vi "Edit VI Theme.vi"(10 "VI Refnum":refnum<vi>) -> ()   [LabVIEW 2021]
doc: "This VI will be the user interface function for the Quick Drop action or through the Tools Menu .\n\nIt will list: +\n- Theme File referenced by the VI (if saved as part of the User Tag data) +\n- Theme Mode referenced by the VI (if saved) +\n- Front Panel Color Rule +\n- All non-free-label Decorations and their color rules; organized by UID because that is the exposed property that is an identifier +\n- All controls on the front panel along with their Color Rules, Boolean Types (if applicable), and Tab Color (if applicable). This will be populated before showing its front panel and will give the user faster access to edit all controls on the front panel. +\n\n->Apply Deocration Rules to see the application of the change +\n->Apply Color Rules to see the application of changes to the controls on the FP +\n->Save VI in order to save all tag data (including theme file and mode reference) +\n\n<b>Code Developed By:</b> +\nDaniel Coons +\nTechnology Service Corporation +\nwww.tsc.com/atcs"
uses:
  Material Theme/Material Theme.lvclass
  _theme-editor/Theme Config/Theme Config.lvclass/Theme Config.ctl
  Material SubVIs/Material SubVIs.lvlib
  user32.dll
  _theme-editor/Theme Config/Theme Config.lvclass
  Quick Drop Plugins/TSC Control Theme Application.llb/control info--typedef.ctl
  Quick Drop Plugins/TSC Control Theme Application.llb/decorations info--typedef.ctl
panel:
  in  "decroation--apply":bool
  in  "decorations":T1[](array[typedef]) {"Decoration Level" items=["Undefined", "Default", "Surface", "Background", "Surface Dim", "Surface Variant", "Surface Bright", "Surface Container Lowest", "Surface Container Low", "Surface Container", "Surface Container High", "Surface Container Highest", "Inverse Surface"]}
  in  "Front Panel Rule":u16(ring) items=["Undefined", "Default", "Surface", "Background", "Surface Dim", "Surface Variant", "Surface Bright", "Surface Container Lowest", "Surface Container Low", "Surface Container", "Surface Container High", "Surface Container Highest", "Inverse Surface"]
  in  "Material Theme":refnum<class "Material Theme.lvclass">
  in  "Close":bool
  in  "save":bool
  in  "Theme Mode":u16(ring) items=["Light", "Light Medium Contrast", "Light High Contrast", "Dark", "Dark Medium Contrast", "Dark High Contrast"]
  in  "Path to theme file":path
  out "Name of VI":string
  in  "apply":bool
  out "header":bool
  in  "Controls":T2[](array[typedef]) {"tab level" items=["Undefined", "N/A", "Default", "Primary Container", "Secondary Container", "Tertiary Container", "Error Container", "Surface", "Background", "Surface Dim", "Surface Variant", "Surface Bright", "Surface Container Lowest", "Surface Container Low", "Surface Container", "Surface Container High", "Surface Container Highest", "Inverse Surface", "Inverse Primary"]; "Boolean Type" items=["Undefined", "N/A", "Outline", "No-Outline", "Tonal", "Filled", "Transparent", "FAB", "Elevated"]; "UI Theme Level" items=["Undefined", "N/A", "Primary", "Secondary", "Tertiary", "Error", "Primary Fixed", "Secondary Fixed", "Tertiary Fixed", "Label Only", "No Change"]}
  # "Decoration UID"
  # "Decoration Color Rule"
  # "Control Name"
  # "Data Type"
  # "Color Rule"
  # "Boolean Type"
  # "Tab Color"
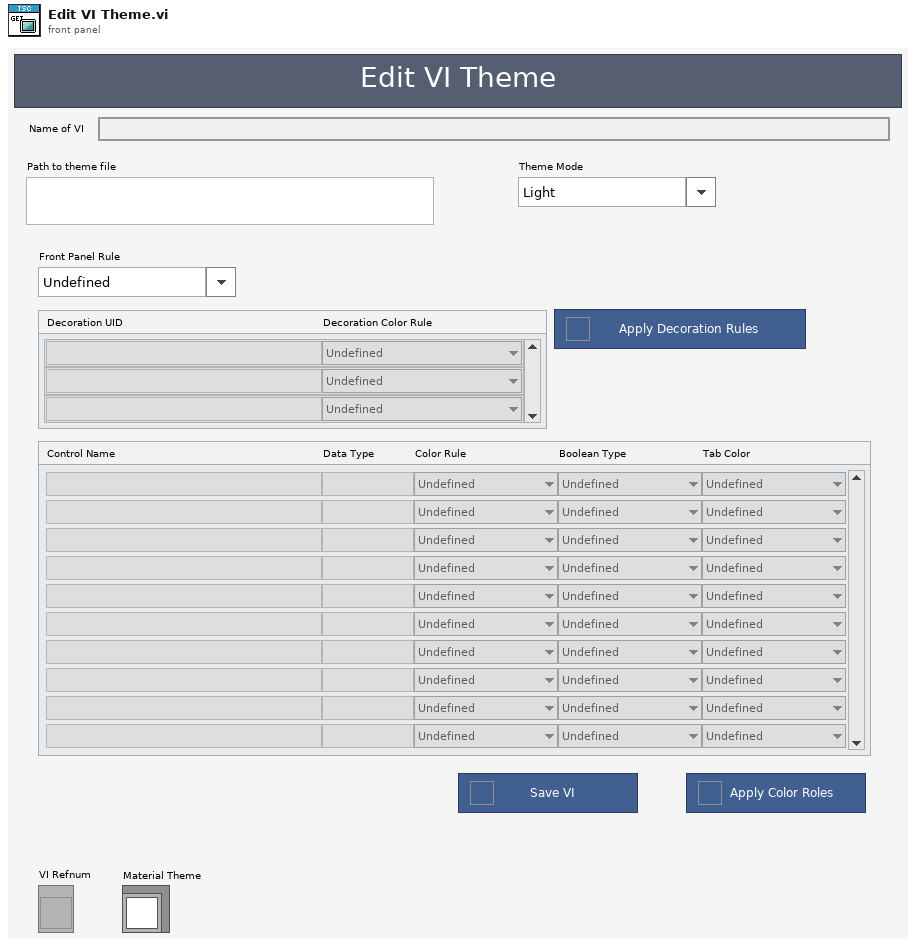
[diagram p1: front panel]
types:
  T1 = typedef "decorations info--typedef.ctl" = cluster{"label":string, "Decoration Level":u16}
  T2 = typedef "control info--typedef.ctl" = cluster{"label":string, "control type":string, "UI Theme Level":u16, "Boolean Type":u16, "tab level":u16}
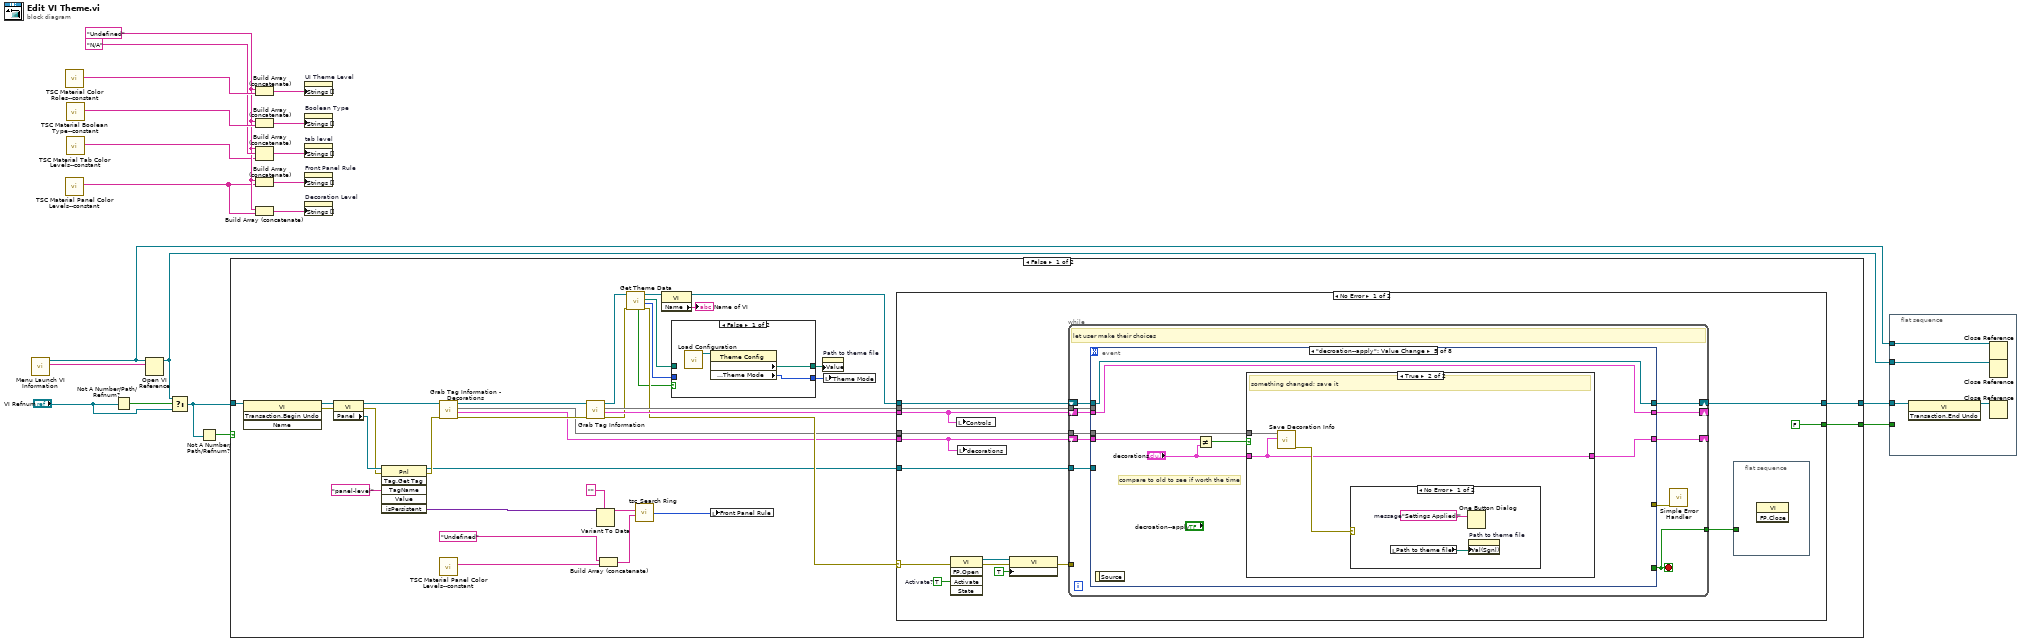
[diagram p0: block diagram]
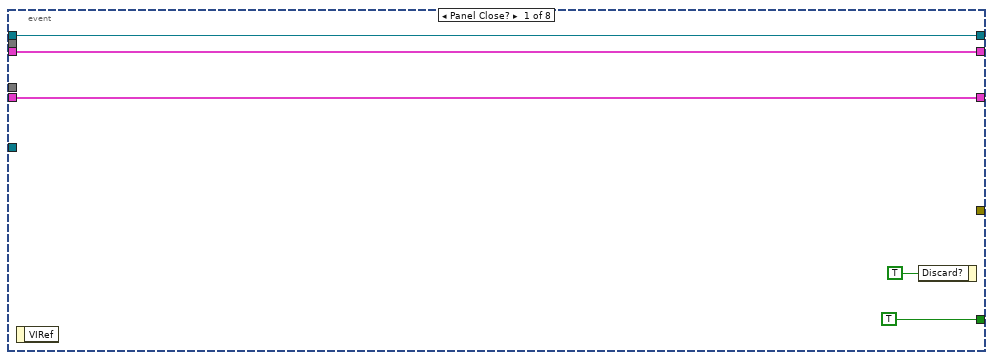
[diagram p3: hidden frame]
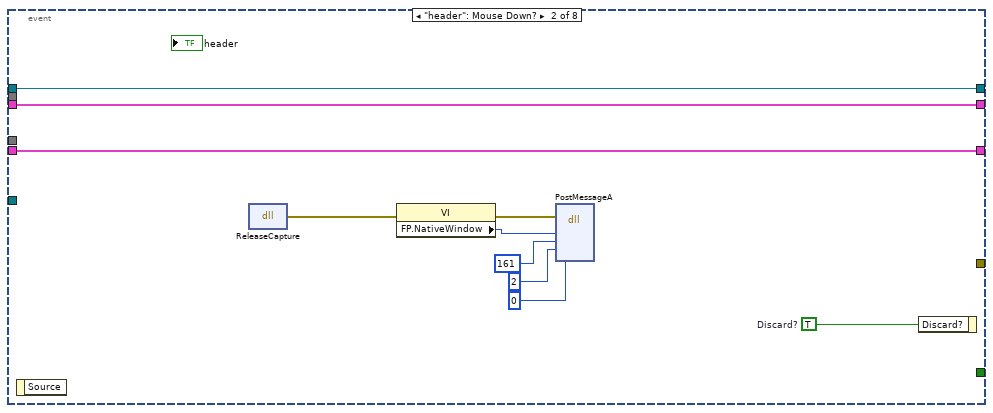
[diagram p4: hidden frame]
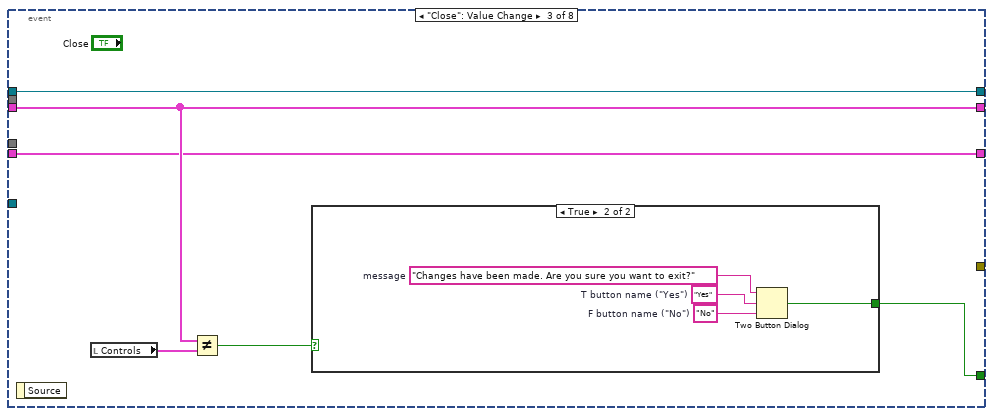
[diagram p5: hidden frame]
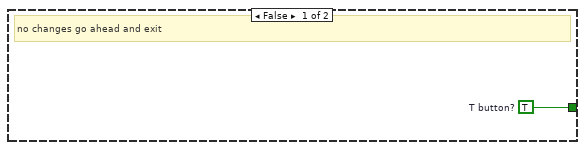
[diagram p6: hidden frame]
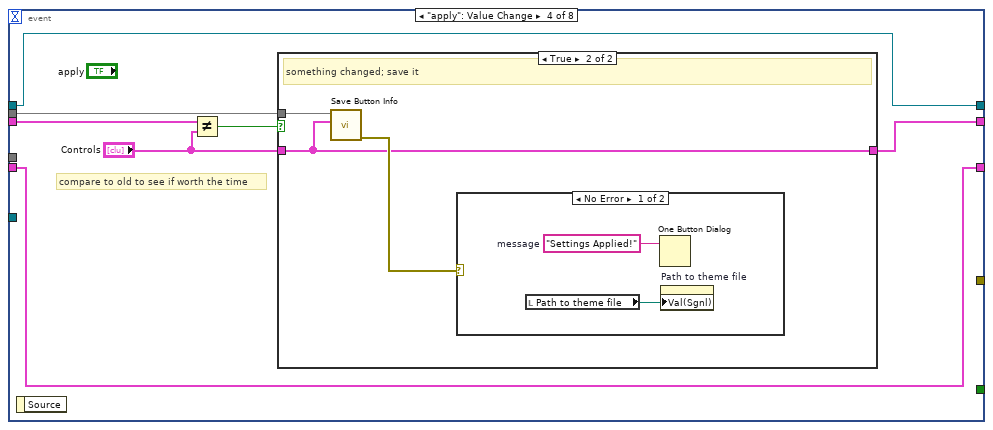
[diagram p7: hidden frame]
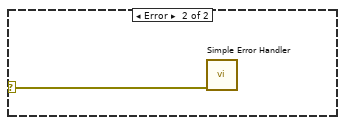
[diagram p9: hidden frame]
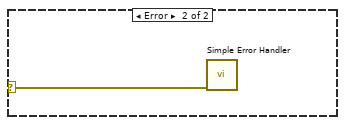
[diagram p11: hidden frame]
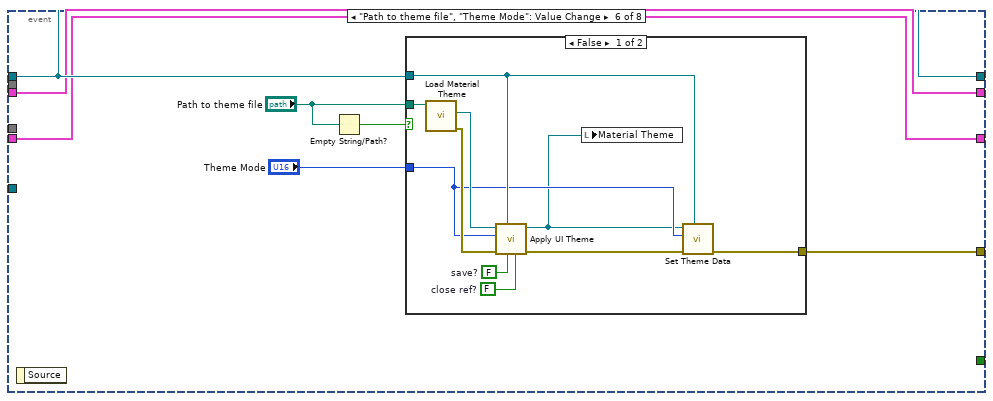
[diagram p12: hidden frame]
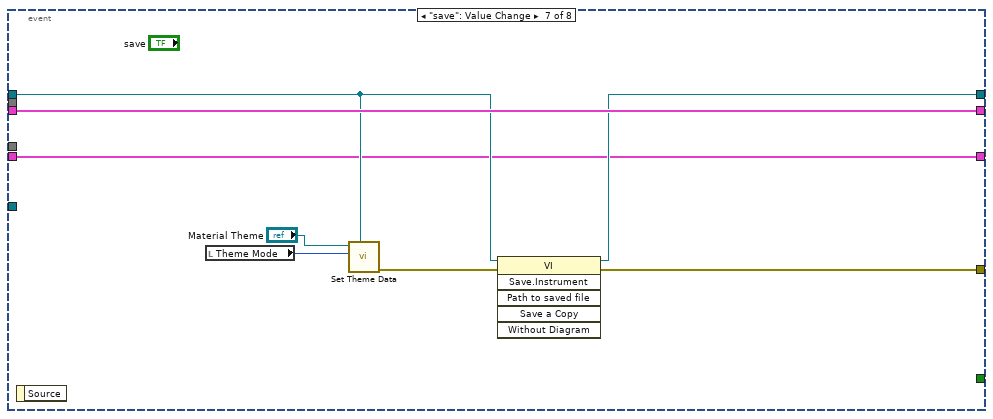
[diagram p14: hidden frame]
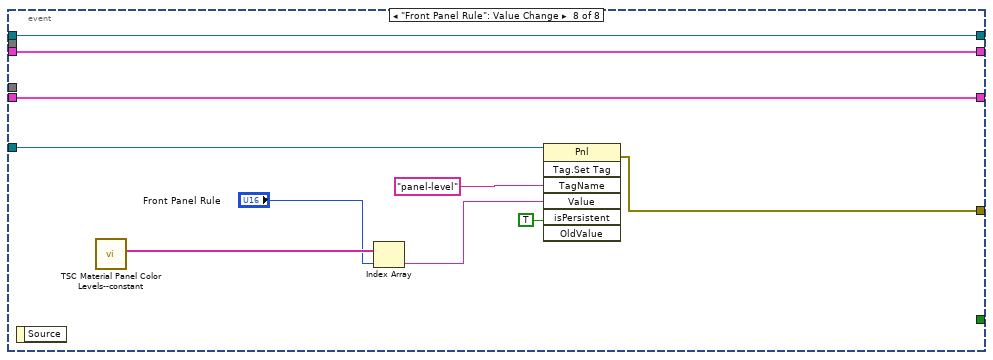
[diagram p15: hidden frame]
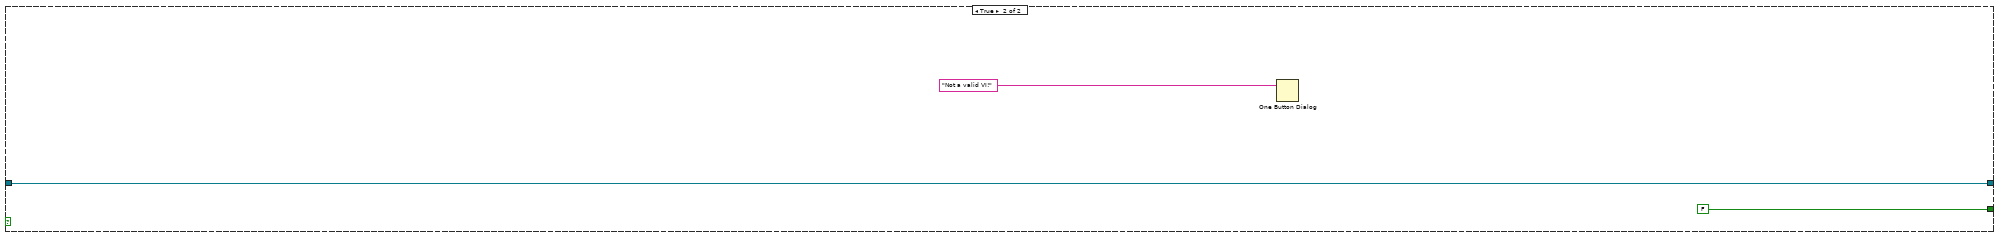
[diagram p17: hidden frame]
diagram:
  w5 = "Undefined"
  n1 = call <vilib>:"Menu Launch VI Information.vi"() -> ("Menu Launch:VI"=w18:string, "Menu Launch:App"=w16:refnum<vi>)  [unwired: 9 in, 1 out]
  n2 = call "TSC Material Color Roles--constant.vi"() -> ("Control Color Roles"=w20:string[])  [unwired: 11 in]
  n3 = call "TSC Material Panel Color Levels--constant.vi"() -> ("front panel color levels"=w2:string[])  [unwired: 11 in]
  n4 = call "TSC Material Boolean Type--constant.vi"() -> ("boolean types"=w9:string[])  [unwired: 11 in]
  n5 = call "TSC Material Tab Color Levels--constant.vi"() -> ("tab color levels"=w3:string[])  [unwired: 11 in]
  n6 = Not A Number/Path/Refnum?(number/path/refnum="VI Refnum") -> (NaN/Path/Refnum?=w19:bool)
  n7 = Open VI Reference(application reference (local)=w16, vi path=w18) -> (vi reference=w15:refnum<vi>)  [unwired: 4 in, 1 out]
  n8 = Select(t=w15, s=w19, f="VI Refnum") -> (s? t:f=w11:refnum<vi>)
  n9 = Not A Number/Path/Refnum?(number/path/refnum=w11) -> (NaN/Path/Refnum?=w10:bool)
  n10 = case shown="False" w10 {
    tunnel: [w54 FALSE] -> w17
    tunnel: w11 -> [w51 w179]
    tunnel: [w39 w179] -> w12
    frame False {
      n11 = invoke class="VI" method="Transaction.Begin Undo"(reference=w51) -> (reference out=w36:refnum<vi>, error out=w50:errorcluster)  [unwired: 3 in, 2 out]
      n12 = property class="VI"(reference=w36, error in=w50) -> (reference out=w24:refnum<vi>, error out=w34:errorcluster, "Panel"=w35:refnum<vi>)
      n13 = invoke class="Pnl" method="Tag.Get Tag"(reference=w35, error in=w34, "TagName"="panel-level" ("Tag Name")) -> (reference out=w26:refnum<vi>, error out=w33:errorcluster, "isPersistent"=w37:variant)  [unwired: 3 in, 3 out]
      n14 = call "Grab Tag Information - Decorations.vi"("error in"=w33, "VI Ref in"=w24) -> ("error out"=w25:errorcluster, "Control Info"=w21:T1[], "map data"=w22:map{string, refnum<vi>}, "VI Ref out"=w23:refnum<vi>)  [unwired: 6 in]
      n15 = call "TSC Material Panel Color Levels--constant.vi"() -> ("front panel color levels"=w30:string[])  [unwired: 11 in]
      n16 = call "Grab Tag Information.vi"("error in"=w25, "VI Ref in"=w23) -> ("error out"=w49:errorcluster, "Control Info"=w53:T2[], "map data"=w52:map{string, refnum<vi>}, "VI Ref out"=w47:refnum<vi>)  [unwired: 6 in]
      n17 = Variant To Data(type="", Variant=w37) -> (data=w31:string)  [unwired: 1 in, 1 out]
      n18 = Build Array (concatenate)("Undefined", w30) -> (w28:string[])
      n19 = call "Get Theme Data.vi"("error in"=w49, "VI Refnum"=w47) -> ("error out"=w48:errorcluster, "Theme"=w43:u16, "Theme Path"=w42:path, "VI Refnum out"=w46:refnum<vi>, "Found?"=w44:bool)  [unwired: 5 in]
      n20 = call "tsc_Search Ring.vi"("Values"=w28, "Search Item"=w31) -> ("Index"=w29:u16)  [unwired: 2 in]
      n21 = property class="VI"(reference=w46) -> (reference out=w45:refnum<vi>, "Name"=→"Name of VI":string)  [unwired: 1 in, 1 out]
      n22 = case shown="False" w44 {
        tunnel: w42 -> [_ w60]
        tunnel: w43 -> [_ w59]
        tunnel: [w57 w60] -> w41
        tunnel: [w56 w59] -> w40
        frame False {
          n23 = call "Load Configuration.vi"() -> ("Theme Config out"=w58:refnum<class "Theme Config.lvclass">)  [unwired: 10 in, 1 out]
          n24 = property class="Theme Config"(reference=w58) -> ("data member access:theme path"=w57:path, "data member access:Theme Mode"=w56:u16)  [unwired: 1 in, 2 out]
        }
        frame True {
        }
      }
      n25 = local write "Front Panel Rule"(w29) -> ()
      n26 = property on="Path to theme file" class="Path"("Value"=w41) -> ()  [unwired: 2 in, 2 out]
      n27 = local write "Theme Mode"(w40) -> ()
      n28 = case shown="No Error" w48 {
        selector: w48 -> [w74 _]
        tunnel: w53 -> [w68 _]
        tunnel: w52 -> [w75 _]
        tunnel: w45 -> [w70 w176]
        tunnel: [FALSE _] -> w54
        tunnel: [w64 w176] -> w39
        tunnel: w26 -> [w63 _]
        tunnel: w22 -> [w62 _]
        tunnel: w21 -> [w61 _]
        frame No Error {
          w73 = TRUE  # Activate?
          n29 = invoke class="VI" method="FP.Open"(error in=w74, "Activate"=w73) -> (reference out=w66:refnum<vi>, error out=w72:errorcluster)  [unwired: 3 in, 3 out]
          n30 = local write "Controls"(w68) -> ()
          n31 = local write "decorations"(w61) -> ()
          n32 = property class="VI"(reference=w66, error in=w72, "Front Panel.IsFrontmost"=TRUE ("Front Panel Window:Is Frontmost")) -> (error out=w67:errorcluster)  [unwired: 1 out]
          n33 = while {
            tunnel: w75 -> [w85]
            tunnel: w67 -> [_]
            tunnel: [w83] -> w71
            shift-right: [w82] -> _
            shift-left: w68 -> [w86]
            shift-right: [w81] -> w64
            shift-left: w70 -> [w84]
            tunnel: w63 -> [w79]
            tunnel: w62 -> [w78]
            shift-right: [w76] -> _
            shift-left: w61 -> [w77]
            stop <- w83 stop-if-true
            # "let user make their choices"
            n34 = event shown="[4] \"decroation--apply\": Value Change" {
              selector: _ -> [_ _ _ _ _ _ _ _]
              dyn-events: _ -> [_ _ _ _ _ _ _ _]
              timeout: _ -> [_ _ _ _ _ _ _ _]
              tunnel: [TRUE _ w105 _ _ _ _ _] -> w83
              tunnel: w86 -> [w89 w94 w104 w119 w129 w143 w165 w175]
              tunnel: w85 -> [_ _ _ w118 _ _ _ _]
              tunnel: w84 -> [w88 w93 w103 w116 w132 w144 w161 w174]
              tunnel: [w89 w94 w104 w114 w129 w143 w165 w175] -> w82
              tunnel: [w88 w93 w103 w116 w132 w144 w164 w174] -> w81
              tunnel: [_ _ _ _ _ w142 w163 w167] -> w80
              tunnel: w79 -> [_ _ _ _ _ _ _ w172]
              tunnel: w78 -> [_ _ _ _ w128 _ _ _]
              tunnel: w77 -> [w87 w92 w102 w113 w130 w141 w158 w166]
              tunnel: [w87 w92 w102 w113 w127 w141 w158 w166] -> w76
              event Panel Close? {
                n35 = event-data() -> ()  [unwired: 1 in, 1 out]
                n36 = event-data("Discard?"=TRUE) -> ()  [unwired: 1 in, 1 out]
              }
              event "header": Mouse Down? {
                w95 = TRUE  # Discard?
                n37 = event-data() -> ()  [unwired: 1 in, 1 out]
                n38 = dll-call lib="user32.dll" fn="ReleaseCapture"() -> (error out=w98:errorcluster)  [unwired: 4 in, 1 out]
                n39 = property class="VI"(error in=w98) -> (error out=w97:errorcluster, "FP.NativeWindow"=w96:u64)  [unwired: 1 in, 1 out]
                n40 = dll-call lib="user32.dll" fn="PostMessageA"(error in=w97, "hWnd"=w96, "Msg"=161, "wParam"=2, "lParam"=0) -> ()  [unwired: 7 in, 2 out]
                n41 = event-data("Discard?"=w95) -> ()  [unwired: 1 in, 1 out]
              }
              event "Close": Value Change {
                n42 = event-data() -> ()  [unwired: 1 in, 1 out]
                n43 = local read "Controls"() -> (w107:T2[])
                n44 = Not Equal?(x=w104, y=w107) -> (x != y?=w106:bool)
                n45 = case shown="True" w106 {
                  tunnel: [w108 w109] -> w105
                  frame False {
                    w108 = TRUE  # T button?
                    # "no changes go ahead and exit"
                  }
                  frame True {
                    w112 = "No"  # F button name ("No")
                    w111 = "Yes"  # T button name ("Yes")
                    w110 = "Changes have been made. Are you sure you want to exit?"  # message
                    n46 = Two Button Dialog(message=w110, 1:w112, 2:w111) -> (T button?=w109:bool)
                  }
                }
              }
              event "apply": Value Change {
                # "compare to old to see if worth the time"
                n47 = event-data() -> ()  [unwired: 1 in, 1 out]
                n48 = Not Equal?(x=w119, y="Controls") -> (x != y?=w117:bool)
                n49 = case shown="True" w117 {
                  tunnel: w118 -> [_ w123]
                  tunnel: "Controls" -> [w120 w121]
                  tunnel: [w120 w121] -> w114
                  frame False {
                    # "no changes"
                  }
                  frame True {
                    # "something changed; save it"
                    n50 = call "Save Button Info.vi"("control info"=w121, "map in"=w123) -> ("error out"=w122:errorcluster)  [unwired: 9 in]
                    n51 = case shown="No Error" w122 {
                      selector: w122 -> [_ w126]
                      frame No Error {
                        w125 = "Settings Applied!"  # message
                        n52 = local read "Path to theme file"() -> (w124:path)
                        n53 = One Button Dialog(message=w125) -> ()  [unwired: 1 in, 1 out]
                        n54 = property on="Path to theme file" class="Path"("Val(Sgnl)"=w124) -> ()  [unwired: 2 in, 2 out]
                      }
                      frame Error {
                        n55 = call <vilib>:"Simple Error Handler.vi"("error in (no error)"=w126) -> ()  [unwired: 4 in, 5 out]
                      }
                    }
                  }
                }
              }
              event "decroation--apply": Value Change {
                # "compare to old to see if worth the time"
                n56 = event-data() -> ()  [unwired: 1 in, 1 out]
                n57 = Not Equal?(x=w130, y="decorations") -> (x != y?=w133:bool)
                n58 = case shown="True" w133 {
                  tunnel: "decorations" -> [w134 w136]
                  tunnel: [w134 w136] -> w127
                  tunnel: w128 -> [_ w135]
                  frame False {
                    # "no changes"
                  }
                  frame True {
                    # "something changed; save it"
                    n59 = call "Save Decoration Info.vi"("control info"=w136, "map in"=w135) -> ("error out"=w137:errorcluster)  [unwired: 9 in]
                    n60 = case shown="No Error" w137 {
                      selector: w137 -> [_ w140]
                      frame No Error {
                        w139 = "Settings Applied!"  # message
                        n61 = local read "Path to theme file"() -> (w138:path)
                        n62 = One Button Dialog(message=w139) -> ()  [unwired: 1 in, 1 out]
                        n63 = property on="Path to theme file" class="Path"("Val(Sgnl)"=w138) -> ()  [unwired: 2 in, 2 out]
                      }
                      frame Error {
                        n64 = call <vilib>:"Simple Error Handler.vi"("error in (no error)"=w140) -> ()  [unwired: 4 in, 5 out]
                      }
                    }
                  }
                }
              }
              event "Path to theme file", "Theme Mode": Value Change {
                n65 = event-data() -> ()  [unwired: 1 in, 1 out]
                n66 = Empty String/Path?(string/path="Path to theme file") -> (empty?=w147:bool)
                n67 = case shown="False" w147 {
                  tunnel: "Path to theme file" -> [w157 _]
                  tunnel: w144 -> [w150 _]
                  tunnel: [w151 _] -> w142
                  tunnel: "Theme Mode" -> [w149 _]
                  frame False {
                    w153 = FALSE  # save?
                    w154 = FALSE  # close ref?
                    n68 = call "Load Material Theme.vi"("file path"=w157) -> ("error out"=w155:errorcluster, "Theme"=w156:refnum<class "Material Theme.lvclass">)  [unwired: 8 in, 1 out]
                    n69 = call "Apply UI Theme.vi"("close ref?"=w154, "save?"=w153, "VI Refnum"=w150, "error in"=w155, "Theme Mode"=w149, "Material Theme in"=w156) -> ("error out"=w152:errorcluster, "Material Theme out"=w148:refnum<class "Material Theme.lvclass">)  [unwired: 4 in]
                    n70 = local write "Material Theme"(w148) -> ()
                    n71 = call "Set Theme Data.vi"("VI Refnum"=w150, "error in"=w152, "Theme"=w149, "Material Theme.lvclass"=w148) -> ("error out"=w151:errorcluster)  [unwired: 7 in]
                  }
                  frame True {
                  }
                }
              }
              event "save": Value Change {
                n72 = event-data() -> ()  [unwired: 1 in, 1 out]
                n73 = local read "Theme Mode"() -> (w160:u16)
                n74 = call "Set Theme Data.vi"("VI Refnum"=w161, "Theme"=w160, "Material Theme.lvclass"="Material Theme") -> ("error out"=w162:errorcluster)  [unwired: 8 in]
                n75 = invoke class="VI" method="Save.Instrument"(reference=w161, error in=w162) -> (reference out=w164:refnum<vi>, error out=w163:errorcluster)  [unwired: 4 in, 4 out]
              }
              event "Front Panel Rule": Value Change {
                n76 = event-data() -> ()  [unwired: 1 in, 1 out]
                n77 = call "TSC Material Panel Color Levels--constant.vi"() -> ("front panel color levels"=w171:string[])  [unwired: 11 in]
                n78 = Index Array(array=w171, index="Front Panel Rule") -> (element=w169:string)
                n79 = invoke class="Pnl" method="Tag.Set Tag"(reference=w172, "TagName"="panel-level" ("Tag Name"), "Value"=w169, "isPersistent"=TRUE ("Is Persistent?")) -> (error out=w167:errorcluster)  [unwired: 3 in, 6 out]
              }
            }
            n80 = call <vilib>:"Simple Error Handler.vi"("error in (no error)"=w80) -> ()  [unwired: 4 in, 5 out]
          }
          n81 = flat-sequence {
            tunnel: w71 -> [_]
            frame #0 {
              n82 = invoke class="VI" method="FP.Close"() -> ()  [unwired: 3 in, 3 out]
            }
          }
        }
        frame Error {
        }
      }
    }
    frame True {
      n83 = One Button Dialog(message="Not a valid VI!") -> ()  [unwired: 1 in, 1 out]
    }
  }
  n84 = Build Array (concatenate)(w5, w20) -> (w13:string[])
  n85 = Build Array (concatenate)(w5, w9) -> (w14:string[])
  n86 = Build Array (concatenate)(w5, "N/A", w3) -> (w7:string[])
  n87 = Build Array (concatenate)(w5, w2) -> (w6:string[])
  n88 = Build Array (concatenate)(w5, w2) -> (w4:string[])
  n89 = property on="UI Theme Level" class="Ring (strict)"("Strings []"=w13) -> ()  [unwired: 2 in, 2 out]
  n90 = property on="Boolean Type" class="Ring (strict)"("Strings []"=w14) -> ()  [unwired: 2 in, 2 out]
  n91 = property on="tab level" class="Ring (strict)"("Strings []"=w7) -> ()  [unwired: 2 in, 2 out]
  n92 = property on="Front Panel Rule" class="Ring (strict)"("Strings []"=w6) -> ()  [unwired: 2 in, 2 out]
  n93 = property on="Decoration Level" class="Ring (strict)"("Strings []"=w4) -> ()  [unwired: 2 in, 2 out]
  n94 = flat-sequence {
    tunnel: w17 -> [_]
    tunnel: w16 -> [w183]
    tunnel: w15 -> [w182]
    tunnel: w12 -> [w181]
    frame #0 {
      n95 = invoke class="VI" method="Transaction.End Undo"(reference=w181) -> (reference out=w180:refnum<vi>)  [unwired: 2 in, 2 out]
      n96 = Close Reference(reference=w183) -> ()  [unwired: 1 in, 1 out]
      n97 = Close Reference(reference=w182) -> ()  [unwired: 1 in, 1 out]
      n98 = Close Reference(reference=w180) -> ()  [unwired: 1 in, 1 out]
    }
  }
